vi "write_attributes.vi"(8 "error in (no error)":errorcluster, 10 "attributes":T1, 11 "TruncatedSVD in":refnum<class "TruncatedSVD.lvclass">) -> (0 "error out":errorcluster, 3 "TruncatedSVD out":refnum<class "TruncatedSVD.lvclass">)   [LabVIEW 2020, in "TruncatedSVD.lvclass"]
uses:
  TruncatedSVD.lvclass
  Controls/truncated_svd_attributes.ctl
  TruncatedSVD.lvclass/TruncatedSVD.ctl
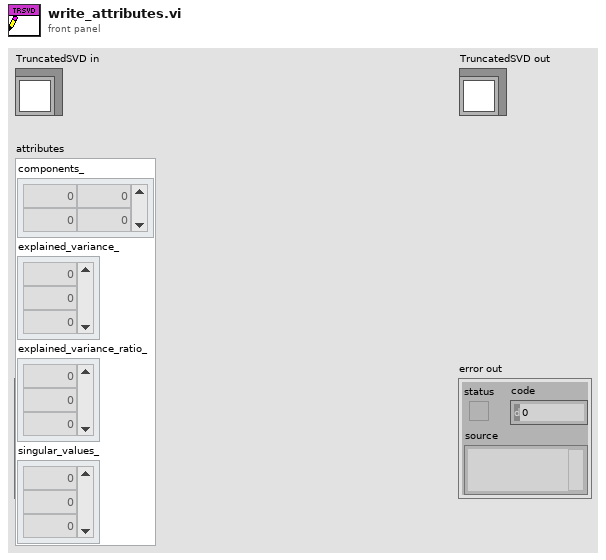
[diagram p1: front panel]
types:
  T1 = typedef "truncated_svd_attributes.ctl" = cluster{"components_":dbl[][], "explained_variance_":dbl[], "explained_variance_ratio_":dbl[], "singular_values_":dbl[]}
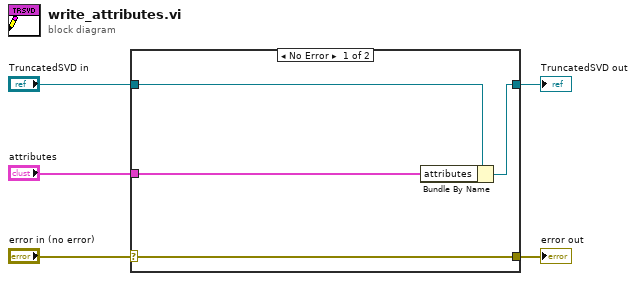
[diagram p0: block diagram]
diagram:
  n1 = case shown="No Error" "error in (no error)" {
    selector: "error in (no error)" -> [w9 w10]
    tunnel: [w9 w10] -> w4
    tunnel: [w7 w11] -> w2
    tunnel: "TruncatedSVD in" -> [w8 w11]
    tunnel: "attributes" -> [w6 _]
    frame No Error {
      n2 = Bundle By Name(cluster=w8, "attributes"=w6) -> (w7:refnum<class "TruncatedSVD.lvclass">)
    }
    frame Error {
    }
  }
  "error out" <- w4
  "TruncatedSVD out" <- w2
